vi "DFD M-Band Cosine-Modulated Filter Bank Design.vi"(4 "weight":dbl=0.5, 5 "signal reconstruction":u16(ring) items=["NPR", "PR"], 6 "fs in [Hz]":dbl=1.0, 7 "band counts":i32=4, 8 "error in (no error)":errorcluster, 10 "roll off":dbl=0.2, 11 "order":i32=39) -> (0 "error out":errorcluster, 3 "filter bank out":T1 {"mFBank_SynthesisFilters"."mMRate_SumWl" min=1 max=32 step=1; "mFBank_SynthesisFilters"."mMRate_InputIwl" min=1 max=32 step=1; "mFBank_SynthesisFilters"."mMRate_GainWl" min=1 max=32 step=1; "mFBank_SynthesisFilters"."mMRate_OutputWl" min=1 max=32 step=1; "mFBank_SynthesisFilters"."mMRate_InputWl" min=1 max=32 step=1; "mFBank_SynthesisFilters"."mMRate_CoefWl" min=1 max=32 step=1; "mFBank_SynthesisFilters"."mMRate_Mode" items=["Default"=-1, "No Rate Change"=0, "Interpolation"=1, "Decimation"=2, "Interpolated"=3, "Rational"=4]; "mFBank_AnalysisFilters"."mMRate_SumWl" min=1 max=32 step=1; "mFBank_AnalysisFilters"."mMRate_InputIwl" min=1 max=32 step=1; "mFBank_AnalysisFilters"."mMRate_GainWl" min=1 max=32 step=1; "mFBank_AnalysisFilters"."mMRate_OutputWl" min=1 max=32 step=1; "mFBank_AnalysisFilters"."mMRate_InputWl" min=1 max=32 step=1; "mFBank_AnalysisFilters"."mMRate_CoefWl" min=1 max=32 step=1; "mFBank_AnalysisFilters"."mMRate_Mode" items=["Default"=-1, "No Rate Change"=0, "Interpolation"=1, "Decimation"=2, "Interpolated"=3, "Rational"=4]; "mFBank_Type" items=["Uniform", "Non-Uniform"]})   [LabVIEW 2017, in "NI_DigFilter_FilterBank.lvlib"]
doc: "Creates an M-band cosine-modulated filter bank."
uses:
  <vilib>/addons/Digital Filter Design/NI_DigFilter_FilterBank.lvlib
  <vilib>/addons/Digital Filter Design/FilterBank.llb/Object/DFD Filter Bank Obj.ctl
  <vilib>/addons/Digital Filter Design/_Objects.llb/DFD Multirate Filter Obj.ctl
  <vilib>/addons/Digital Filter Design/_Objects.llb/DFD Multirate Mode.ctl
  <vilib>/addons/Digital Filter Design/_Objects.llb/DFD Coef Norm Type.ctl
  <vilib>/addons/Digital Filter Design/_Objects.llb/DFD Round-off Mode.ctl
  <vilib>/addons/Digital Filter Design/_Objects.llb/DFD FXP MRate Multiply Mode.ctl
  <vilib>/addons/Digital Filter Design/FilterBank.llb/Object/DFD Filter Bank Processing Method.ctl
  <vilib>/addons/Digital Filter Design/FilterBank.llb/Object/DFD Filter Bank Type.ctl
  <vilib>/addons/Digital Filter Design/NI_DigFilterLicensed.lvlib
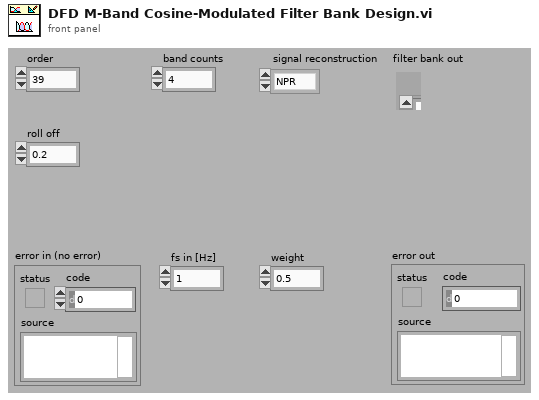
[diagram p1: front panel]
types:
  T1 = typedef "NI_DigFilter_FilterBank.lvlib/DFD Filter Bank Obj.ctl" = cluster{"mFBank_AnalysisFilters":T2[], "mFBank_SynthesisFilters":T2[], "mFBank_#Bands":i32, "mFBank_ProcMethod":T7, "mFBank_Coeffs":dbl[], "mFBank_Gain":dbl, "mFBank_Delay":i32, "mFBank_Type":T8}
  T2 = typedef "NI_DigFilterLicensed.lvlib/DFD Multirate Filter Obj.ctl" = cluster{"mMRate_Structure":enum16{"CIC", "FIR", "IIR", "Lattice"}, "mMRate_Mode":T3, "mMRate_Factor":i32, "mMRate_FIRParams":cluster{"mMRate_FIR_H":dbl[], "mMRate_FIR_IsNyquist?":bool, "mMRate_FIR_IsSymmetric?":bool}, "mMRate_CICParams":cluster{"mMRate_CIC_#Stage":i32, "mMRate_CIC_Lag":i32, "mMRate_CIC_Type":enum16{"Lowpass", "Highpass"}}, "mMRate_Order":i32, "mMRate_Version":string, "mMRate_Comments":string, "mMRate_RationalFactor":cluster{"mMRate_L":i32, "mMRate_M":i32}, "mMRate_Fs":dbl, "mMRate_Quantized?":bool, "mMRate_QFilterGain":dbl, "mMRate_CoefWl":i16, "mMRate_Scaling":cluster{"mMRate_ScaleByPowerOf2?":bool, "mMRate_ScaleType":T4}, "mMRate_InputWl":i16, "mMRate_OutputWl":i16, "mMRate_OutputMode":T5, "mMRate_MultMode":T6, "mMRate_BitPruning":bool, "mMRate_GainWl":i16, "mMRate_OutputFwl":i16, "mMRate_SumIwl":i16, "mMRate_InputIwl ":i16, "mMRate_SumWl":i16, "mMRate_CoefIwl":i16}
  T3 = typedef "NI_DigFilterLicensed.lvlib/DFD Multirate Mode.ctl" = i16
  T4 = typedef "NI_DigFilterLicensed.lvlib/DFD Coef Norm Type.ctl" = enum16{"No Norm", "Time Domain 1-Norm", "Time Domain 2-Norm", "Time Domain Inf-Norm"}
  T5 = typedef "NI_DigFilterLicensed.lvlib/DFD Round-off Mode.ctl" = enum16{"Nearest", "Truncation"}
  T6 = typedef "NI_DigFilterLicensed.lvlib/DFD FXP MRate Multiply Mode.ctl" = enum16{"Truncated", "Full"}
  T7 = typedef "NI_DigFilter_FilterBank.lvlib/DFD Filter Bank Processing Method.ctl" = enum16{"General", "2-Band QMF Lattice", "Cosine-Modulated"}
  T8 = typedef "NI_DigFilter_FilterBank.lvlib/DFD Filter Bank Type.ctl" = u16
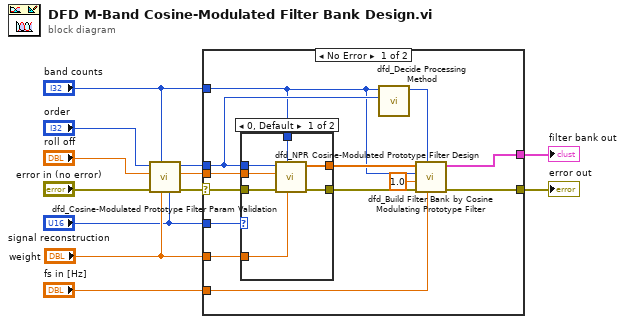
[diagram p0: block diagram]
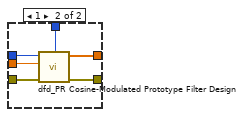
[diagram p2: hidden frame]
diagram:
  n1 = call <vilib>:"dfd_Cosine-Modulated Prototype Filter Param Validation.vi"("PR?"="signal reconstruction", "weight"="weight", "number of bands"="band counts", "error in (no error)"="error in (no error)", "roll off"="roll off", "order"="order") -> ("error out"=w2:errorcluster, "dup roll off"=w4:dbl, "dup order"=w3:i32)  [unwired: 3 in]
  n2 = case shown="No Error" w2 {
    selector: w2 -> [w22 w39]
    tunnel: "weight" -> [w25 _]
    tunnel: "band counts" -> [w18 _]
    tunnel: [w14 w39] -> w7
    tunnel: [w15 _] -> w6
    tunnel: "signal reconstruction" -> [w24 _]
    tunnel: w4 -> [w23 _]
    tunnel: w3 -> [w21 _]
    tunnel: "fs in [Hz]" -> [w16 _]
    frame No Error {
      n3 = case shown="0, Default" w24 {
        tunnel: [w32 w33] -> w17
        tunnel: w25 -> [w31 _]
        tunnel: w22 -> [w30 w35]
        tunnel: w23 -> [w29 w36]
        tunnel: w18 -> [w28 w37]
        tunnel: w21 -> [w27 w38]
        tunnel: [w26 w34] -> w19
        frame 0, Default {
          n4 = call <vilib>:"dfd_NPR Cosine-Modulated Prototype Filter Design.vi"("weight"=w31, "band counts"=w28, "error in (no error)"=w30, "roll off"=w29, "order"=w27) -> ("error out"=w32:errorcluster, "h"=w26:dbl[])  [unwired: 5 in]
        }
        frame 1 {
          n5 = call <vilib>:"dfd_PR Cosine-Modulated Prototype Filter Design.vi"("M"=w37, "error in (no error)"=w35, "roll off"=w36, "order"=w38) -> ("error out"=w33:errorcluster, "h"=w34:dbl[])  [unwired: 6 in]
        }
      }
      n6 = call <vilib>:"dfd_Decide Processing Method.vi"("order"=w21, "band counts"=w18) -> ("processing method"=w20:T7)  [unwired: 9 in]
      n7 = call <vilib>:"dfd_Build Filter Bank by Cosine Modulating Prototype Filter.vi"("fs in [Hz]"=w16, "processing method"=w20, "error in"=w17, "gain"=1.0, "band counts"=w18, "filter coefficients"=w19) -> ("error out"=w14:errorcluster, "filter bank out"=w15:T1)  [unwired: 4 in]
    }
    frame Error {
    }
  }
  "error out" <- w7
  "filter bank out" <- w6
